vi "MtrPowerDigital.vi"(8 "PwrDwn":bool, 9 "PwrUp":bool, 11 "PwrON":bool) -> (3 "MtrPWR":dbl)   [LabVIEW 2015]
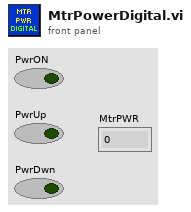
[diagram p1: front panel]
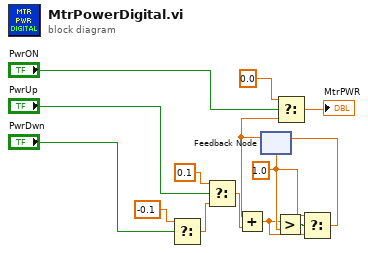
[diagram p0: block diagram]
diagram:
  w7 = 1.0
  n1 = Select(t=-0.1, s="PwrDwn") -> (s? t:f=w10:dbl)  [unwired: 1 in]
  n2 = Select(t=0.1, s="PwrUp", f=w10) -> (s? t:f=w13:dbl)
  n3 = feedback #1(w7) -> (w12:dbl)
  n4 = Add(x=w12, y=w13) -> (x+y=w6:dbl)
  n5 = Greater?(x=w6, y=w7) -> (0:w8:bool)
  n6 = Select(t=0.0 ("Output"), s="PwrON", f=w12) -> (s? t:f=→"MtrPWR":dbl)
  n7 = Select(t=w7, s=w8, f=w6) -> (s? t:f=w5:dbl)
  n8 = feedback-in #1(w5) -> ()
